vi "Read Attribute.vi"(0 "ILinked List in":refnum<class "ILinked List.lvclass">, 1 "Linked List ID":string, 2 "Include Private?":bool, 3 "Flatten Pointer?":bool, 5 "Attribute Name":string, 9 "Type":variant, 11 "error in (no error)":errorcluster) -> (4 "ILinked List out":refnum<class "ILinked List.lvclass">, 6 "Attribute Name out":string, 10 "Attribute":variant, 12 "Found?":bool, 14 "Data ID":string, 15 "error out":errorcluster)   [LabVIEW 2020, in "Linked Lists.lvlib" / "ILinked List.lvclass"]
uses:
  <vilib>/gpm_packages/@cs/linked-list/Source/Linked List/ILinkedList/ILinked List.lvclass
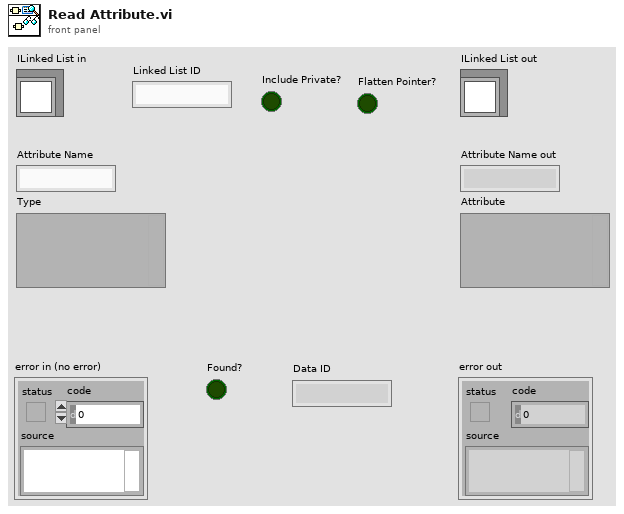
[diagram p1: front panel]
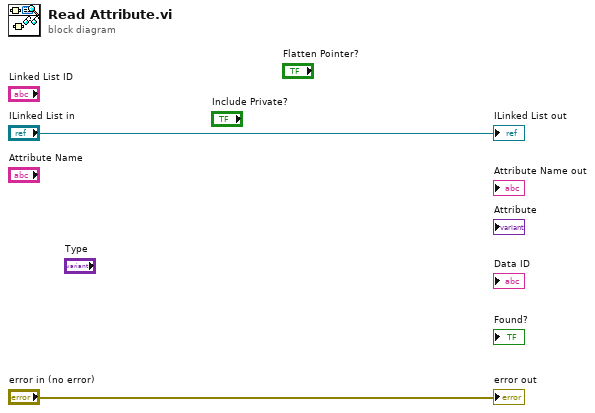
[diagram p0: block diagram]
diagram:
  "error out" <- "error in (no error)"
  "ILinked List out" <- "ILinked List in"
